vi "GetOwningPane.vi"(6 "error in":errorcluster, 9 "Control in":refnum<class "Control.lvclass">) -> (0 "error out":errorcluster, 3 "Control out":refnum<class "Control.lvclass">, 4 "Owning Pane":i32)   [LabVIEW 2014, in "Control.lvclass"]
uses:
  Control.lvclass
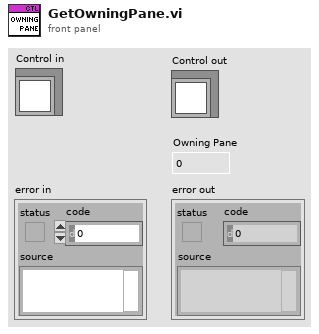
[diagram p1: front panel]
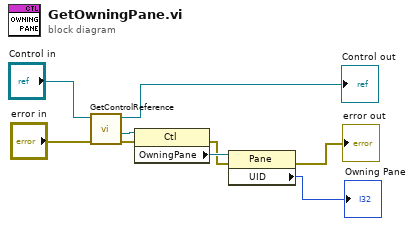
[diagram p0: block diagram]
diagram:
  n1 = call "GetControlReference.vi"("error in"="error in", "Control in"="Control in") -> ("error out"=w6:errorcluster, "control reference"=w7:refnum<vi>, "Control out"=→"Control out":refnum<class "Control.lvclass">)  [unwired: 7 in]
  n2 = property class="Ctl"(reference=w7, error in=w6) -> (error out=w4:errorcluster, "OwningPane"=w5:refnum<vi>)  [unwired: 1 out]
  n3 = property class="Pane"(reference=w5, error in=w4) -> (error out=→"error out":errorcluster, "UID"=→"Owning Pane":i32)  [unwired: 1 out]
